vi "Find Control Ref in Cluster.vi"(8 "error in (no error)":errorcluster, 10 "Control Name":string, 11 "Cluster ref in":refnum<vi>) -> (0 "error out":errorcluster, 1 "Found ?":bool, 2 "Ctl ref":refnum<vi>, 3 "Cluster ref out":refnum<vi>)   [LabVIEW 2019, in "gRPC Scripting Tools.lvlib"]
uses:
  gRPC Scripting Tools.lvlib
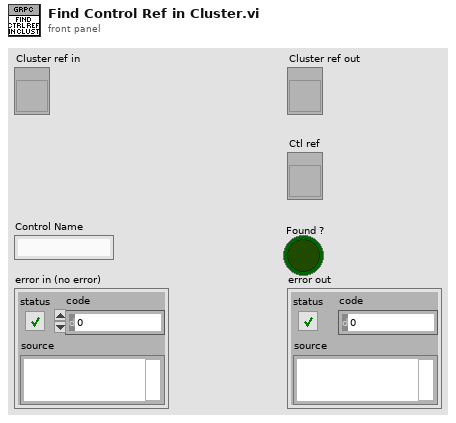
[diagram p1: front panel]
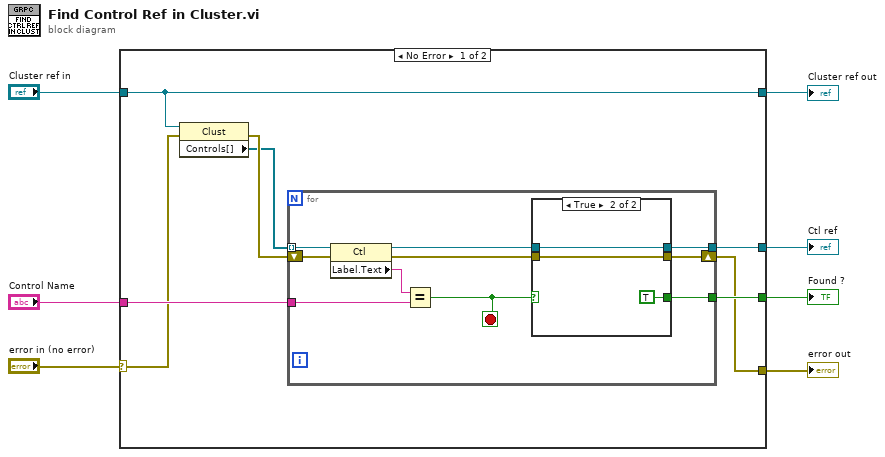
[diagram p0: block diagram]
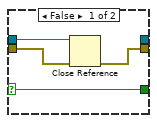
[diagram p2: hidden frame]
diagram:
  n1 = case shown="No Error" "error in (no error)" {
    selector: "error in (no error)" -> [w12 w34]
    tunnel: "Control Name" -> [w13 _]
    tunnel: "Cluster ref in" -> [w11 w33]
    tunnel: [w8 w34] -> w5
    tunnel: [w11 w33] -> w2
    tunnel: [w10 _] -> w3
    tunnel: [w9 _] -> w1
    frame No Error {
      n2 = property class="Clust"(reference=w11, error in=w12) -> (error out=w15:errorcluster, "Controls[]"=w14:refnum<vi>[])  [unwired: 1 out]
      n3 = for {
        tunnel: w14 -> [w25] mode=indexing
        tunnel: w13 -> [w24]
        shift-right: [w18] -> w8
        shift-left: w15 -> [w23]
        tunnel: [w17] -> w10
        tunnel: [w16] -> w9
        stop <- w21 stop-if-true
        n4 = property class="Ctl"(reference=w25, error in=w23) -> (reference out=w20:refnum<vi>, error out=w19:errorcluster, "Label.Text"=w22:string)
        n5 = Equal?(x=w22, y=w24) -> (x = y?=w21:bool)
        n6 = case shown="True" w21 {
          selector: w21 -> [w26 _]
          tunnel: w20 -> [w29 w30]
          tunnel: w19 -> [w28 w32]
          tunnel: [w27 w32] -> w18
          tunnel: [w26 TRUE] -> w17
          tunnel: [_ w30] -> w16
          frame False {
            n7 = Close Reference(reference=w29, error in (no error)=w28) -> (error out=w27:errorcluster)
          }
          frame True {
          }
        }
      }
    }
    frame Error {
    }
  }
  "error out" <- w5
  "Cluster ref out" <- w2
  "Found ?" <- w3
  "Ctl ref" <- w1
